vi "Clear and flush table.vi"(8 "error in":errorcluster, 11 "Trace":refnum<vi>) -> (0 "error out":errorcluster)   [LabVIEW 2025, in "CAN-LIN Raw Bus Capture UI.lvlib"]
uses:
  CAN-LIN Raw Bus Capture UI.lvlib
  <vilib>/Utility/miscctls.llb/LVRowAndColumnTypeDef.ctl
  Flush Table.vi
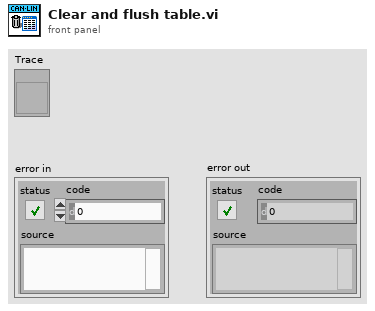
[diagram p1: front panel]
types:
  T1 = typedef "LVRowAndColumnTypeDef.ctl" = cluster{"Row":i32, "Column":i32}
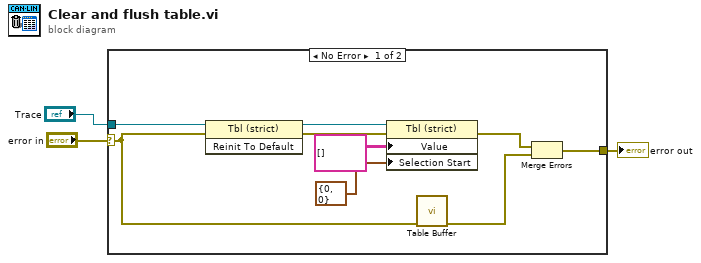
[diagram p0: block diagram]
diagram:
  n1 = case shown="No Error" "error in" {
    selector: "error in" -> [w5 w13]
    tunnel: "Trace" -> [w8 _]
    tunnel: [w4 w13] -> w1
    frame No Error {
      n2 = invoke class="Tbl (strict)" method="Reinit To Default"(reference=w8, error in=w5) -> (reference out=w9:refnum<vi>, error out=w10:errorcluster)  [unwired: 1 in, 1 out]
      n3 = property on="Property Node" class="Tbl (strict)"(reference=w9, error in=w10, "Value"=string[][] [], "Selection Start"=T1 {"Row"=0, "Column"=0}) -> (error out=w7:errorcluster)  [unwired: 1 out]
      n4 = call-poly "Table Buffer.vi"("error in"=w5) -> ("error out"=w6:errorcluster)  [unwired: 10 in]
      n5 = Merge Errors(w7, w6) -> (w4:errorcluster)
    }
    frame Error {
    }
  }
  "error out" <- w1
